vi "AT Wait Buffer A.vi"(8 "error in (no error)":errorcluster, 9 "Input buffer":u64, 10 "Timeout":u32, 11 "Handle":i32) -> (0 "error out":errorcluster, 1 "Output buffer":u64, 2 "PtrSize":i32, 3 "Status":i32)   [LabVIEW 2019]
doc: "Wait Buffer\n\nOutput:\n I32 Status\n U64 Output buffer\n I32 PtrSize\n\nInput:\n I32 Handle\n U64 Input buffer\n U32 Timeout\n \nThis function is used to receive notification whenever a previously queued image buffer contains data. The\naddress of the buffer that is now available is returned in the Ptr parameter. The PtrSize parameter will return\nwith the size of the returned image buffer. The Timeout parameter can be specified to indicate how long in\nmilliseconds you wish to wait for the next available image. The function will put the calling thread to sleep until either an image becomes available or the Timeout elapses."
uses:
  atcoreA.dll
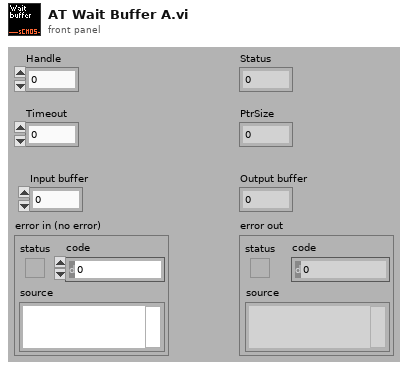
[diagram p1: front panel]
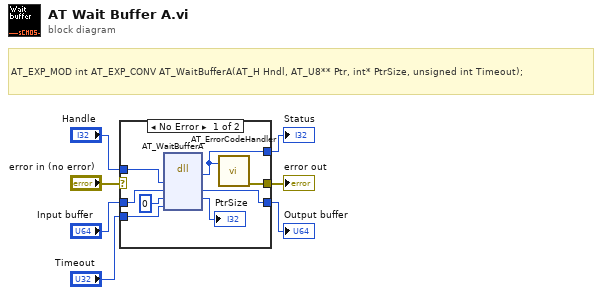
[diagram p0: block diagram]
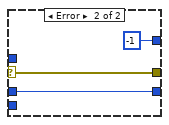
[diagram p2: hidden frame]
diagram:
  # "AT_EXP_MOD int AT_EXP_CONV AT_WaitBufferA(AT_H Hndl, AT_U8** Ptr, int* PtrSize, unsigned int Timeout);"
  n1 = case shown="No Error" "error in (no error)" {
    selector: "error in (no error)" -> [_ w18]
    tunnel: [w8 -1 ("return type")] -> w7
    tunnel: "Handle" -> [w15 _]
    tunnel: "Timeout" -> [w12 _]
    tunnel: [w9 w18] -> w3
    tunnel: "Input buffer" -> [w10 w16]
    tunnel: [w11 w16] -> w2
    frame No Error {
      n2 = dll-call lib="atcoreA.dll" fn="AT_WaitBufferA"("Handle"=w15, "Ptr"=w10, "PtrSize"=0, "Timeout"=w12) -> ("Status"=w8:i32, "Ptr"=w11:u64, "PtrSize"=→"PtrSize":i32)  [unwired: 5 in, 2 out]
      n3 = call <userlib>:"AT_ErrorCodeHandler.vi"("Error"=w8) -> ("error out"=w9:errorcluster)  [unwired: 6 in]
    }
    frame Error {
    }
  }
  "Status" <- w7
  "error out" <- w3
  "Output buffer" <- w2
